vi "Notify.vi"(8 "error in (no error)":errorcluster caption="entrée d'erreur (pas d'erreur)", 9 "Data":variant, 10 "command":T1="DL:finishedmoving", 11 "Message en entrée":refnum<class "Message.lvclass">) -> (0 "error out":errorcluster caption="sortie d'erreur", 3 "Message en sortie":refnum<class "Message.lvclass">)   [LabVIEW 2019, in "Message.lvclass"]
uses:
  Message.lvclass
  dependecies/ControlsVIs/Clusters-def/SERVER-Commands.ctl
  Message.lvclass/Message.ctl
  Control/Control-Server/Control-Server.lvclass
panel:
  in  "attente (ms)":u32=1
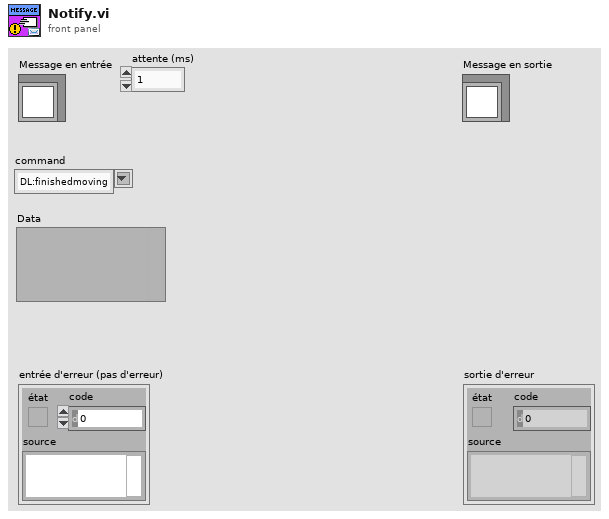
[diagram p1: front panel]
types:
  T1 = typedef "Control-Server.lvclass/SERVER-Commands.ctl" = string
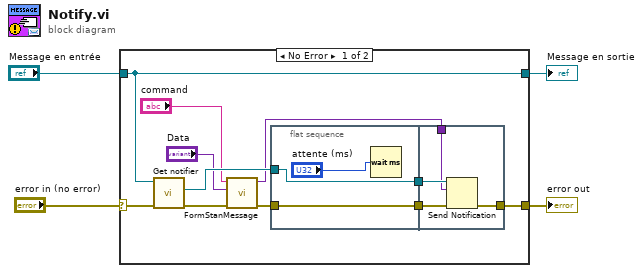
[diagram p0: block diagram]
diagram:
  n1 = case shown="No Error" "error in (no error)" {
    selector: "error in (no error)" -> [w7 w24]
    tunnel: [w13 w24] -> w3
    tunnel: [w15 w23] -> w1
    tunnel: "Message en entrée" -> [w15 w23]
    frame No Error {
      n2 = call "Get notifier.vi"("error in (no error)"=w7, "Message en entrée"=w15) -> ("error out"=w6:errorcluster, "notifier"=w14:refnum<notifier>)  [unwired: 7 in, 1 out]
      n3 = call "FormStanMessage.vi"("error in"=w6, "data"="Data", "Command"="command") -> ("error out"=w5:errorcluster, "message"=w8:variant)  [unwired: 7 in]
      n4 = flat-sequence {
        tunnel: w14 -> [w18]
        tunnel: [w18] -> w12
        tunnel: [w16] -> w11
        tunnel: w5 -> [w16]
        tunnel: [w20] -> w13
        tunnel: w12 -> [w22]
        tunnel: w11 -> [w21]
        tunnel: w8 -> [w19]
        frame #0 {
          n5 = Wait (ms)(milliseconds to wait="attente (ms)") -> ()  [unwired: 1 out]
        }
        frame #1 {
          n6 = Send Notification(notification=w19, notifier=w22, error in (no error)=w21) -> (error out=w20:errorcluster)  [unwired: 1 out]
        }
      }
    }
    frame Error {
    }
  }
  "error out" <- w3
  "Message en sortie" <- w1
